vi "Power ON_OFF.vi"(3 "OFF (T)/ON (F)":bool, 4 "MM System":u16(ring) items=["MM3000", "MM2000"], 5 "PC Bus Address":u32=832 format="%.0x") -> (2 "Error":bool)   [LabVIEW 2022 SP3]
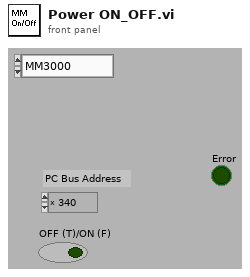
[diagram p1: front panel]
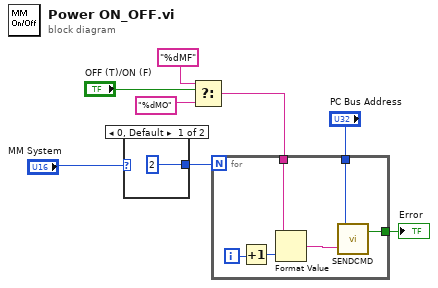
[diagram p0: block diagram]
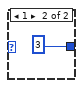
[diagram p2: hidden frame]
diagram:
  n1 = case shown="0, Default" "MM System" {
    tunnel: [2 3] -> w7
    frame 0, Default {
    }
    frame 1 {
    }
  }
  n2 = Select(t="%dMF", s="OFF (T)/ON (F)", f="%dMO") -> (s? t:f=w4:string)
  n3 = for {
    N: w7 -> [_]
    tunnel: "PC Bus Address" -> [w16]
    tunnel: w4 -> [w12]
    tunnel: [w11] -> w2
    i -> [w14]
    n4 = Increment(x=w14) -> (x+1=w13:i32)
    n5 = Format Value(format string=w12, value (0)=w13) -> (output string=w15:string)  [unwired: 1 out]
    n6 = call "SENDCMD.VI"("MM2000 Command (ASCII String)"=w15, "MM2000 Address (Hexadecimal)"=w16) -> ("Boolean"=w11:bool)  [unwired: 1 in]
  }
  "Error" <- w2
